vi "terminate.vi"(8 "error in (no error)":errorcluster, 11 "GenericPlugin in":refnum<class "DataCollectionDL110128Streaming.lvclass">) -> (0 "error out":errorcluster, 3 "GenericPlugin out":refnum<class "DataCollectionDL110128Streaming.lvclass">)   [LabVIEW 2010, in "DataCollectionDL110128Streaming.lvclass"]
doc: "The dynamic dispatch version of this VI terminates the plug-in object by releasing all of its resources."
uses:
  DataCollectionDL110128Streaming.lvclass
  DataCollectionDL110128Streaming.lvclass/DataCollectionDL110128Streaming.ctl
  DataCollectionDL091104Scaffold/DataCollectionDL091104Scaffold/DataCollectionDL091104Scaffold.lvclass
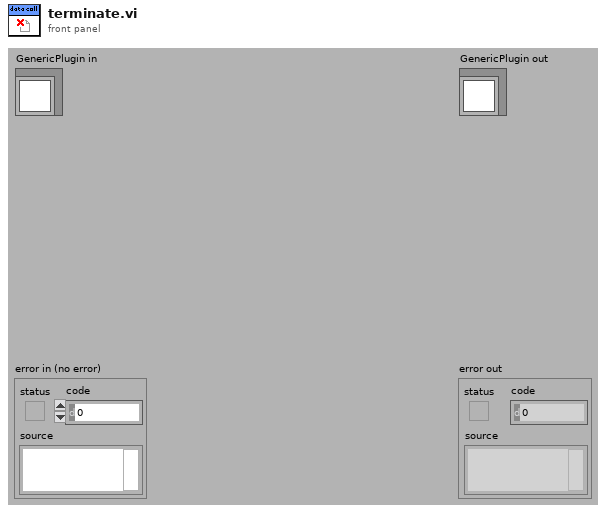
[diagram p1: front panel]
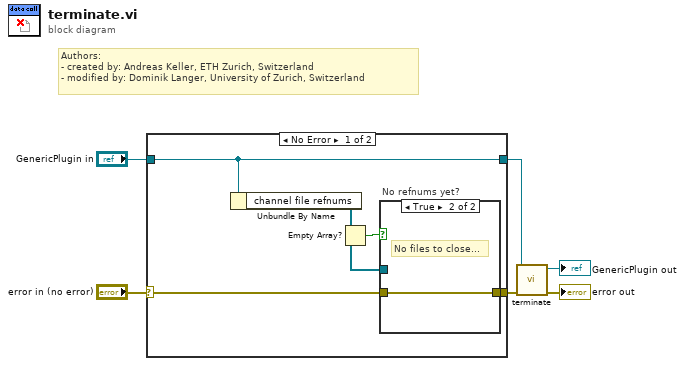
[diagram p0: block diagram]
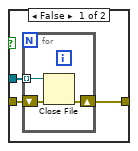
[diagram p2: hidden frame]
diagram:
  # "Authors: \n- created by: Andreas Keller, ETH Zurich, Switzerland\n- modified by: Dominik Langer, University of Zurich, Switzerland"
  n1 = case shown="No Error" "error in (no error)" {
    selector: "error in (no error)" -> [w7 w20]
    tunnel: [w9 w20] -> w4
    tunnel: "GenericPlugin in" -> [w8 w19]
    tunnel: [w8 w19] -> w2
    frame No Error {
      n2 = Unbundle By Name(w8) -> ("channel file refnums"=w10:refnum<file>[])
      n3 = Empty Array?(array=w10) -> (empty?=w11:bool)
      n4 = case "No refnums yet?" shown="True" w11 {
        tunnel: w7 -> [w14 w18]
        tunnel: [w12 w18] -> w9
        tunnel: w10 -> [w13 _]
        frame False {
          n5 = for {
            tunnel: w13 -> [w16] mode=indexing
            shift-right: [w15] -> w12
            shift-left: w14 -> [w17]
            n6 = Close File(refnum=w16, error in=w17) -> (error out=w15:errorcluster)  [unwired: 1 out]
          }
        }
        frame True {
          # "No files to close..."
        }
      }
    }
    frame Error {
    }
  }
  n7 = call-parent "terminate.vi"("error in (no error)"=w4, "GenericPlugin in"=w2) -> ("error out"=→"error out":errorcluster, "GenericPlugin out"=→"GenericPlugin out":refnum<class "DataCollectionDL110128Streaming.lvclass">)  [unwired: 8 in]
